vi "Extract Most Significant Orders (Offline) .vi"() -> ()   [LabVIEW 2017]
doc: "<B>DESCRIPTIONS</B>:\nThis VI demonstrates how to extract the order waveforms of the highest power from a simulated signal or recorded data. The recorded data is acquired with Log Data (Analog Tacho, DAQmx).vi or Log Data (Analog Tacho, Traditional DAQ).vi.\n\n<B>INSTRUCTIONS</B>:\n1. Select the <B>Generate Signal</B> tab to use simulated signal or the <B>Load Data</B> tab to load recorded data.\n2. When using a simulated signal, specify the <B>sampling info</B>, <B>signal rotating speed</B> and <B>order components</B> contained in the signal.\n3. When using recorded data, select the data file to load.\n4. Specify the <B>number of significant orders</B> to extract. Specify the <B>bandwidth</B>, <B>window info</B>, <B>x-axis selection</B>, and <B>view</B> to get the desired display of the order waveforms. \n4. Run the VI.\n5. If you want to view signals of other channels, select the signal of interest in <B>select channel</B>. Run the VI again to make the changes take effect.\n\n<B>ORDER ANALYSIS VIs USED IN THIS EXAMPLE</B>:\n1. SVL Scale Voltage to EU.vi\n2. OAT Analog Tacho Process.vi\n3. OAT Extract Most Significant Order Waveforms.vi\n4. OAT Order Magnitude and Phase.vi"
uses:
  <vilib>/addons/Sound and Vibration/compatibility/Controls/svl_Channel Info.ctl
  <vilib>/addons/Sound and Vibration/compatibility/Controls/svl_Engineering Units Text Ring.ctl
  <vilib>/addons/Sound and Vibration/compatibility/Controls/svl_Weighting Filter Text Ring.ctl
  <vilib>/addons/Sound and Vibration/Order Analysis/Ref Gabor Order Tracking/Mask Bandwidth.ctl
  <vilib>/addons/Sound and Vibration/svt_Calibration/SVL Scale Voltage to EU (1 Ch).vi
  <vilib>/addons/Sound and Vibration/svt_Calibration/SVL Scale Voltage to EU (N Ch - N Info).vi
  <vilib>/addons/_NISVFA/_Shared subVIs/Common/svc_Set SV Channel Info.vi
  <vilib>/addons/_NISVFA/_Shared subVIs/Common/svc_Set SV Channel Info (variant).vi
  <vilib>/addons/_NISVFA/_Shared subVIs/Common/SVL Set dB Reference (variant).vi
  <vilib>/addons/Sound and Vibration/Order Analysis/Gabor Order Tracking/OAT Order Magnitude and Phase (Order Waveforms).vi
  <vilib>/addons/Sound and Vibration/Order Analysis/Tach Process/OAT Analog Tacho Process (1 Tacho).vi
  <vilib>/addons/_NISVFA/_Shared subVIs/Common/svc_Caller VI Returned in Error Source.vi
  <vilib>/addons/_NISVFA/_Shared subVIs/Common/svc_Engineering Units to Unit Label.vi
  <vilib>/addons/_NISVFA/_Shared subVIs/Common/svc_Set dB ref if Pascal.vi
  <vilib>/addons/_NISVFA/_Shared subVIs/Common/svc_Compute Scale Factor to Convert C to EU.vi
  <vilib>/addons/_NISVFA/_Shared subVIs/Common/svc_Compute Scale Factor to Convert V to EU.vi
  <vilib>/addons/Sound and Vibration/svt_Calibration/SoundVib_Calibration.lvlib
  <vilib>/addons/Sound and Vibration/Order Analysis/Tach Process/SoundVib_TachProcess.lvlib
  <vilib>/addons/Sound and Vibration/Order Analysis/Gabor Order Tracking/SoundVib_Gabor.lvlib
  <vilib>/addons/Sound and Vibration/Order Analysis/Resample Order Tracking/SoundVib_OrderTracking.lvlib
panel:
  in  "select channel":u16(ring) items=["channel 1"]
  in  "view":T1={"dB on? (F)"=FALSE, "unwrap phase? (T)"=TRUE, "unit in degree? (T)"=TRUE}
  in  "windows info":cluster{"window type":u32, "window length":i32}={"window type"=62, "window length"=2048} {"window length" min=2; "window type" items=["None"=0, "Hanning"=1, "Hamming"=2, "Blackman-Harris"=3, "Exact Blackman"=4, "Blackman"=5, "Flat Top"=6, "4 Term B-Harris"=7, "7 Term B-Harris"=8, "Low Sidelobe"=9, "Gaussian"=62]}
  in  "X axis selection":u16(ring) items=["Time", "Revolution", "RPM"]
  in  "bandwidth":T2={"bandwidth value"=0.5, "bandwidth unit"=enum."Order"} {"bandwidth value" min=0.0 format="%.2f"}
  out "significant orders":dbl[](array[numeric])=[1.0] format="%.2f"
  in  "number of significant orders":i32=3
  in  "Tab Control 2":enum32{"Generate Signal", "Load Data"}(tab)
  in  "channel info":T3={"sensor sensitivity [mV/EU]"=1000.0, "engineering units"=1, "dB reference [EU]"=1.0, "custom label"="EU", "weighting filter"=0, "pregain [dB]"=0.0} {"pregain [dB]" format="%.2f"; "weighting filter" items=["Linear", "A-weighting", "B-weighting", "C-weighting", "ITU-R 468-4", "Dolby", "CCITT", "C-message"]; "dB reference [EU]" format="%^.1e"; "engineering units" items=["custom..."=0, "V"=1, "A"=21, "Pa"=2, "N"=20, "g"=3, "m/s^2"=4, "m/s"=5, "m"=6, "mm/s"=12, "mm"=13, "microns/s"=14, "microns"=15, "in/s^2"=7, "in/s"=8, "in"=9, "mils/s"=10, "mils"=11, "rad/s^2"=16, "rad/s"=17, "rad"=18, "strain"=19]; "sensor sensitivity [mV/EU]" format="%.2f"}
  in  "order components":T6(array[cluster])=[{"order"=1, "amplitude"=1.0, "phase (deg)"=0.0, "order envelop"=0}, {"order"=2, "amplitude"=0.5, "phase (deg)"=0.0, "order envelop"=2}, {"order"=3, "amplitude"=0.25, "phase (deg)"=0.0, "order envelop"=1}, {"order"=10, "amplitude"=1.0, "phase (deg)"=0.0, "order envelop"=2}] {"order envelop" items=["None", "Sine", "Triangle"]}
  in  "sampling info":T7={"sampling frequency"=10000.0, "duration [s]"=10.0} {"sampling frequency" format="%#_6p"}
  in  "signal rotating speed":u16(ring)=3 items=["3000 RPM", "1000-6000 RPM", "6000-1000 RPM", "1000-6000-1000 RPM"]
  in  "Data Path":path
  out "fs":dbl=44100.0
  out "number of samples":i32=44100
  in  "Tab Control":T8(tab)
  out "speed profile":T9(graph)
  out "vibration signals":waveform(dbl)[](graph)
  out "phase":T10(graph)
  out "magnitude":T10(graph)
  # "Select Help»Show Context Help and move the cursor over the VI icon for more information."
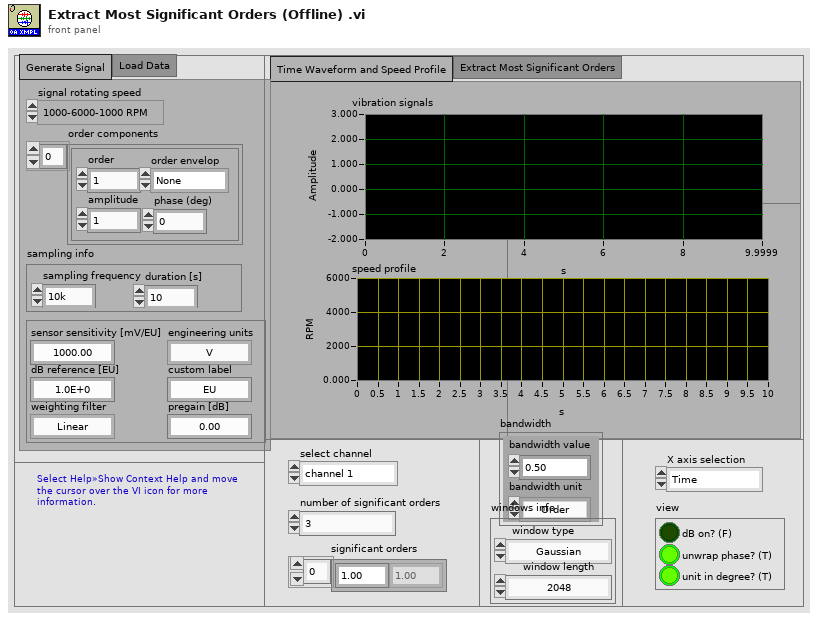
[diagram p1: front panel]
types:
  T1 = cluster{"dB on? (F)":bool, "unwrap phase? (T)":bool, "unit in degree? (T)":bool}
  T2 = typedef "SoundVib_Gabor.lvlib/Mask Bandwidth.ctl" = cluster{"bandwidth value":dbl, "bandwidth unit":enum16{"Order", "Hz"}}
  T3 = typedef "svl_Channel Info.ctl" = cluster{"sensor sensitivity [mV/EU]":dbl, "engineering units":T4, "dB reference [EU]":dbl, "custom label":string, "weighting filter":T5, "pregain [dB]":dbl}
  T4 = typedef "svl_Engineering Units Text Ring.ctl" = u16
  T5 = typedef "svl_Weighting Filter Text Ring.ctl" = u16
  T6 = cluster{"order":i32, "amplitude":dbl, "phase (deg)":dbl, "order envelop":u16}[]
  T7 = cluster{"sampling frequency":dbl, "duration [s]":dbl}
  T8 = enum32{"Time Waveform and Speed Profile", "Extract Most Significant Orders"}
  T9 = typedef "SoundVib_TachProcess.lvlib/speed profile.ctl" = cluster{"time [s]":dbl[], "speed [RPM]":dbl[]}
  T10 = cluster{"time/rev/rpm":dbl[], "magnitude":dbl[]}[]
  T11 = typedef "svc_Channel Info.ctl" = cluster{"sensor sensitivity":dbl, "engineering units":T12, "dB reference":dbl, "custom label":string, "weighting filter":T13, "pregain":dbl}
  T12 = typedef "svc_Engineering Units Text Ring.ctl" = u16
  T13 = typedef "svc_Weighting Filter Text Ring.ctl" = u16
  T14 = cluster{"pulse / rev":i32, "threshold (auto)":dbl, "slope (Rising)":u16}
  T15 = typedef "SoundVib_Gabor.lvlib/window information.ctl" = cluster{"window type":u32, "window length":i32}
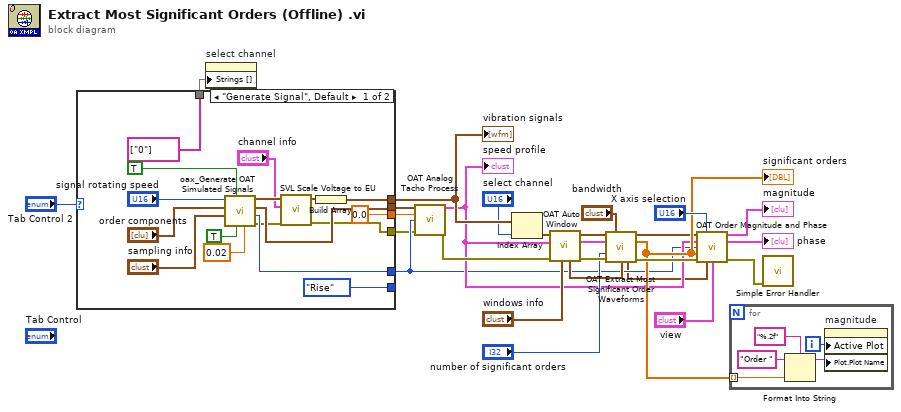
[diagram p0: block diagram]
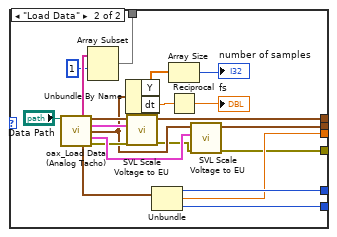
[diagram p2: hidden frame]
diagram:
  n1 = case shown="\"Generate Signal\", Default" "Tab Control 2" {
    tunnel: [w38 w59] -> w24
    tunnel: [w35 w53] -> w26
    tunnel: [w34 w57] -> w6
    tunnel: [enum16{"Rise", "Fall"}."Rise" ("slope (Rise)") w56] -> _
    tunnel: [0.0 ("threshold (auto)") w55] -> w25
    tunnel: [string[] ["0"] w47] -> w2
    tunnel: [w28 w45] -> w1
    frame "Generate Signal", Default {
      n2 = call <vilib>:"oax_Generate OAT Simulated Signals.vi"("noise level"=0.02, "add noise?"=TRUE, "reset?"=TRUE, "sampling info"="sampling info", "ordercomponents"="order components", "signal rotating speed"="signal rotating speed") -> ("error out"=w33:errorcluster, "pulse/revolution"=w34:i32, "Tach Signal"=w35:waveform(dbl), "Vibration Signal"=w37:waveform(dbl))  [unwired: 2 in]
      n3 = call-poly <vilib>:"SVL Scale Voltage to EU.vi"("error in (no error)"=w33, "channel info"="channel info", "signal [V]"=w37) -> ("error out"=w28:errorcluster, "scaled signal [EU]"=w36:waveform(dbl))  [unwired: 6 in, 1 out]
      n4 = Build Array(w36) -> (w38:waveform(dbl)[])
    }
    frame "Load Data" {
      n5 = call <vilib>:"oax_Load Data (Analog Tacho).vi"("Data Path In"="Data Path") -> ("channel name"=w49:string[], "vibration data"=w60:waveform(dbl)[], "vibration channel info"=w51:T11[], "analog tacho signal"=w50:waveform(dbl), "tacho channel info"=w54:T11, "tacho info"=w58:T14, "error out"=w52:errorcluster)  [unwired: 8 in]
      n6 = Array Subset(array=w49, index=1) -> (w47:string[])  [unwired: 1 in]
      n7 = Unbundle By Name(w50) -> ("Y"=w62:dbl[], "dt"=w64:dbl)
      n8 = call-poly <vilib>:"SVL Scale Voltage to EU.vi"("error in (no error)"=w52, "channel info"=w51, "signals [V]"=w60) -> ("error out"=w46:errorcluster, "scaled signals [EU]"=w59:waveform(dbl)[])  [unwired: 6 in, 1 out]
      n9 = Unbundle(w58) -> ("pulse / rev"=w57:i32, "threshold (auto)"=w55:dbl, "slope (Rising)"=w56:u16)
      n10 = Array Size(array=w62) -> (size(s)=→"number of samples":i32)
      n11 = Reciprocal(x=w64) -> (1/x=→"fs":dbl)
      n12 = call-poly <vilib>:"SVL Scale Voltage to EU.vi"("error in (no error)"=w46, "channel info"=w54, "signal [V]"=w50) -> ("error out"=w45:errorcluster, "scaled signal [EU]"=w53:waveform(dbl))  [unwired: 6 in, 1 out]
    }
  }
  "vibration signals" <- w24
  n13 = property on="select channel" class="Ring (strict)"("Strings []"=w2) -> ()  [unwired: 2 in, 2 out]
  n14 = call-poly <vilib>:"OAT Analog Tacho Process.vi"("analog tacho signal"=w26, "threshold (auto)"=w25, "pulse/revolution (1)"=w6, "error in (no error)"=w1) -> ("speed profile"=w7:T9, "error out"=w17:errorcluster)  [unwired: 7 in, 3 out]
  "speed profile" <- w7
  n15 = Index Array(array=w24, index="select channel") -> (element=w18:waveform(dbl))
  n16 = call <vilib>:"OAT Auto Window.vi"("window info in"="windows info", "error in (no error)"=w17, "speed profile"=w7, "scaled signal [EU]"=w18) -> ("error out"=w21:errorcluster, "speed profile out"=w19:T9, "scaled signal [EU] out"=w23:waveform(dbl), "window info out"=w22:T15)  [unwired: 4 in]
  n17 = call <vilib>:"OAT Extract Most Significant Order Waveforms.vi"("scaled signal [EU]"=w23, "speed profile"=w19, "number of orders (3)"="number of significant orders", "error in (no error)"=w21, "bandwidth"="bandwidth", "window info"=w22) -> ("order waveforms [EU]"=w8:waveform(dbl)[], "orders"=w9:dbl[], "actual window info"=w5:T15, "error out"=w20:errorcluster)  [unwired: 5 in, 1 out]
  "significant orders" <- w9
  n18 = call-poly <vilib>:"OAT Order Magnitude and Phase.vi"("order waveforms [EU]"=w8, "x-axis selection"="X axis selection", "speed profile"=w7, "pulse/revolution (1)"=w6, "orders to compute (1.0)"=w9, "error in (no error)"=w20, "window info"=w5, "view"="view") -> ("magnitudes [RMS]"=→"magnitude":T10, "phases [phase lag]"=→"phase":cluster{"time/rev/rpm":dbl[], "phase":dbl[]}[], "error out"=w14:errorcluster)  [unwired: 2 in, 3 out]
  n19 = for {
    tunnel: w9 -> [w70] mode=indexing
    i -> [w67]
    n20 = Format Into String(format string="%.2f" ("Format String"), initial string="Order " ("Input String"), w70) -> (resulting string=w66:string)  [unwired: 1 in, 1 out]
    n21 = property on="magnitude" class="XYGraph (strict)"("Active Plot"=w67, "Plot.Plot Name"=w66) -> ()  [unwired: 2 in, 2 out]
  }
  n22 = call <vilib>:"Simple Error Handler.vi"("error in (no error)"=w14) -> ()  [unwired: 4 in, 5 out]
